vi "Configure Session.vi"(8 "error in":errorcluster, 11 "Plugin in":refnum<class "FFT.lvclass">) -> (0 "error out":errorcluster, 3 "Plugin out":refnum<class "FFT.lvclass">)   [LabVIEW 2024, in "FFT.lvlib" / "FFT.lvclass"]
uses:
  FFT.lvclass
  C:/Program Files/National Instruments/LabVIEW 2024/vi.lib/FlexLogger/SDK/PluginSDK.lvlibp/PEFClasses/SDK/Plugin/Plugin.lvclass
  FFT.lvclass/FFT.ctl
  FFT Globals.vi
  <vilib>/FlexLogger/SDK/PluginSDK.lvlibp/PEFClasses/SDK/Plugin/ParameterAccess/Read Boolean.vi
  <vilib>/FlexLogger/SDK/PluginSDK.lvlibp/PEFClasses/SDK/Plugin/ParameterAccess/Read I32.vi
  <vilib>/FlexLogger/SDK/PluginSDK.lvlibp/PEFClasses/SDK/Plugin/ParameterAccess/Write I32.vi
  <vilib>/FlexLogger/SDK/PluginSDK.lvlibp/PEFClasses/SDK/Plugin/Plugin.lvclass
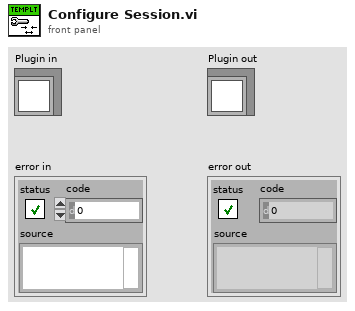
[diagram p1: front panel]
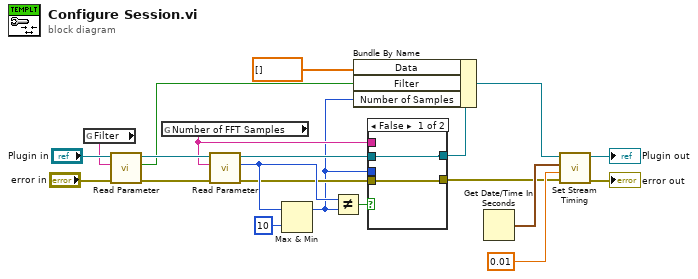
[diagram p0: block diagram]
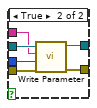
[diagram p2: hidden frame]
diagram:
  n1 = global read "FFT Globals.vi" "Filter"() -> (w14:string)
  n2 = call-poly <vilib>:"Read Parameter.vi"("error in (no error)"="error in", "Name"=w14, "Plugin in"="Plugin in") -> ("error out"=w10:errorcluster, "Value"=w11:bool, "Plugin out"=w13:refnum<class "FFT.lvclass">)  [unwired: 5 in, 1 out]
  n3 = global read "FFT Globals.vi" "Number of FFT Samples"() -> (w3:string)
  n4 = call-poly <vilib>:"Read Parameter.vi"("error in (no error)"=w10, "Name"=w3, "Plugin in"=w13) -> ("error out"=w4:errorcluster, "Value"=w8:i32, "Plugin out"=w7:refnum<class "FFT.lvclass">)  [unwired: 5 in, 1 out]
  n5 = Max & Min(x=w8, y=10) -> (max(x,y)=w2:i32)  [unwired: 1 out]
  n6 = Not Equal?(x=w8, y=w2) -> (x != y?=w5:bool)
  n7 = case shown="False" w5 {
    tunnel: w7 -> [w23 w29]
    tunnel: [w23 w28] -> w6
    tunnel: w4 -> [w22 w27]
    tunnel: w3 -> [_ w26]
    tunnel: w2 -> [_ w25]
    tunnel: [w22 w24] -> w1
    frame False {
    }
    frame True {
      n8 = call-poly <vilib>:"Write Parameter.vi"("error in (no error)"=w27, "Value"=w25, "Name"=w26, "Plugin in"=w29) -> ("error out"=w24:errorcluster, "Plugin out"=w28:refnum<class "FFT.lvclass">)  [unwired: 6 in]
    }
  }
  n9 = Bundle By Name(cluster=w6, "Data"=dbl[] [], "Filter"=w11, "Number of Samples"=w2) -> (w12:refnum<class "FFT.lvclass">)
  n10 = Get Date/Time In Seconds() -> (seconds since 1Jan1904=w19:timestamp)
  n11 = call-dynamic "Set Stream Timing.vi"("error in (no error)"=w1, "dt(sec)"=0.01, "Start Time"=w19, "Plugin in"=w12) -> ("error out"=→"error out":errorcluster, "Plugin out"=→"Plugin out":refnum<class "FFT.lvclass">)  [unwired: 6 in]
